vi "local variable.vi"() -> ()   [LabVIEW 2025]
panel:
  out "Boolean":bool
  in  "milliseconds to wait 3":u32
  out "String 3":string
  out "Numeric 3":dbl
  out "Loop3":bool
  in  "Numeric 2":dbl
  in  "Switch 2":bool
  in  "String 2":string
  in  "milliseconds to wait 2":u32
  out "Loop3":bool
  out "Loop 2":bool
  in  "milliseconds to wait":u32
  out "Loop 1":bool
  in  "String":string
  in  "Switch":bool
  in  "Numeric":dbl
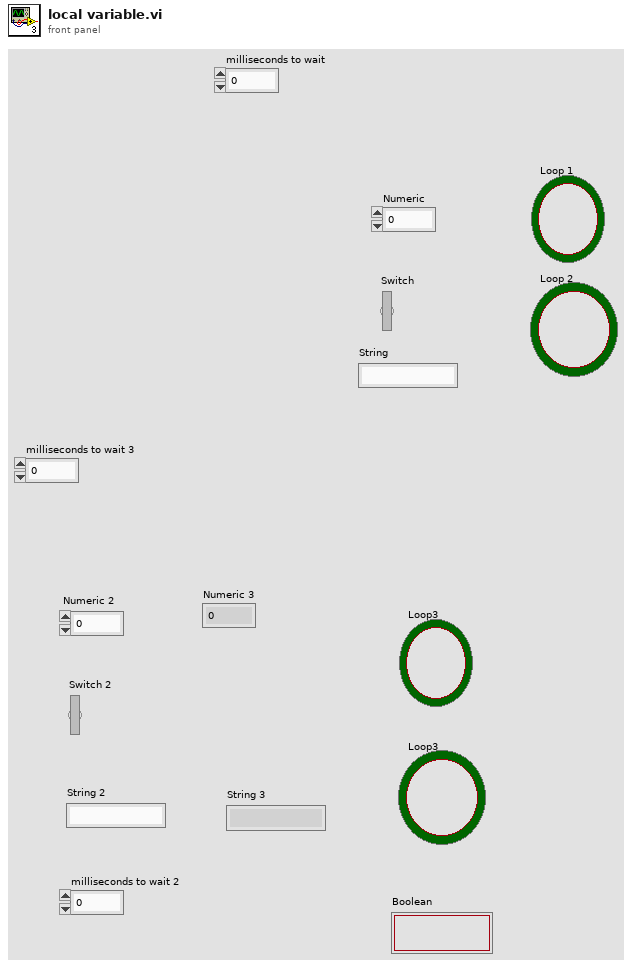
[diagram p1: front panel]
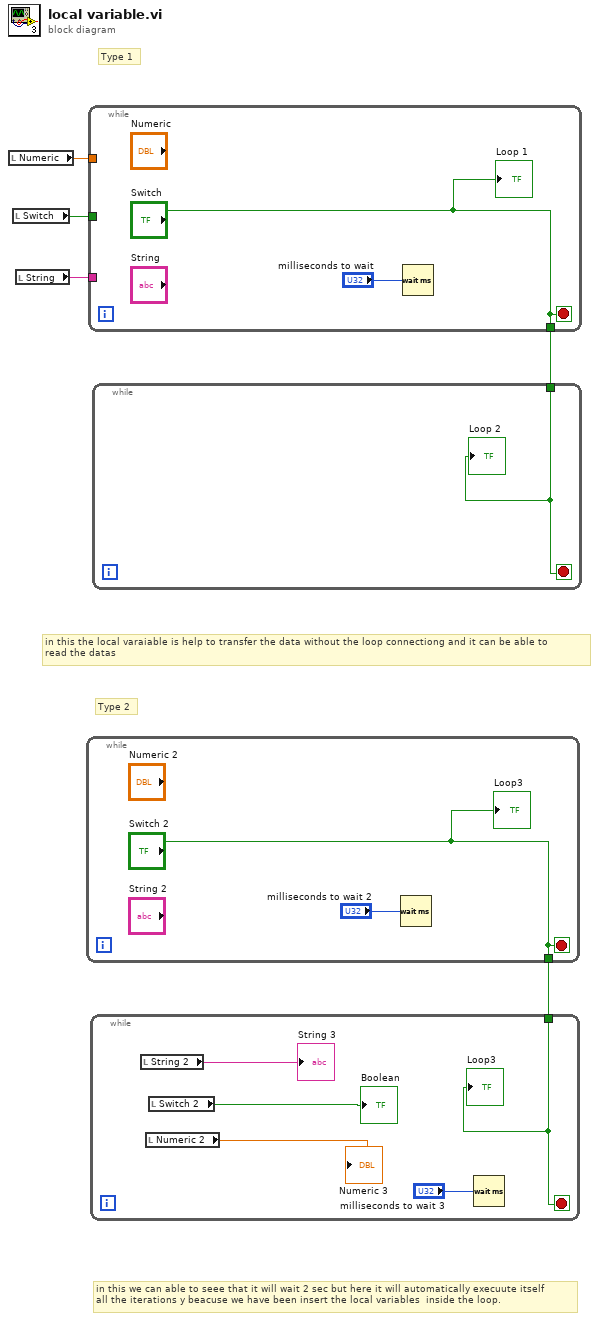
[diagram p0: block diagram]
diagram:
  # "in this we can able to seee that it will wait 2 sec but here it will automatically execuute itself \nall the iterations y beacuse we have been insert the local variables  inside the loop."
  # "Type 1"
  # "Type 2"
  # "in this the local varaiable is help to transfer the data without the loop connectiong and it can be able to \nread the datas"
  n1 = local read "Numeric"() -> (w5:dbl)
  n2 = local read "Switch"() -> (w4:bool)
  n3 = local read "String"() -> (w3:string)
  n4 = while {
    tunnel: ["Switch 2"] -> w1
    stop <- "Switch 2" stop-if-true
    n5 = Wait (ms)(milliseconds to wait="milliseconds to wait 2") -> ()  [unwired: 1 out]
    "Loop3" <- "Switch 2"
  }
  n6 = while {
    tunnel: w5 -> [_]
    tunnel: [w9] -> _
    tunnel: w4 -> [w9]
    tunnel: w3 -> [_]
    tunnel: ["Switch"] -> w2
    stop <- "Switch" stop-if-true
    n7 = Wait (ms)(milliseconds to wait="milliseconds to wait") -> ()  [unwired: 1 out]
    "Loop 1" <- "Switch"
  }
  n8 = while {
    tunnel: w1 -> [w12]
    stop <- w12 stop-if-true
    n9 = local read "String 2"() -> (→"String 3":string)
    n10 = local read "Numeric 2"() -> (→"Numeric 3":dbl)
    n11 = local read "Switch 2"() -> (→"Boolean":bool)
    n12 = Wait (ms)(milliseconds to wait="milliseconds to wait 3") -> ()  [unwired: 1 out]
    "Loop3" <- w12
  }
  n13 = while {
    tunnel: w2 -> [w16]
    stop <- w16 stop-if-true
    "Loop 2" <- w16
  }
